vi "Group Memory.vi"(8 "error in (no error)":errorcluster, 9 "Group Initialization Set":T3[](array[typedef]), 10 "Group":string, 11 "Method":T5) -> (0 "error out":errorcluster, 1 "Group Indices Out":T4[](array[typedef]), 2 "Tag Sets Out":T1[](array[typedef]), 3 "Tags/Groups Out":string[](array[string]))   [LabVIEW 2016, in "CVT.lvlib" / "Current Value Table.lvlib"]
doc: "This VI stores references to the indices of every tag in each group, sorted by data type."
uses:
  <vilib>/NI/Current Value Table/Current Value Table.lvlib
  <vilib>/NI/Current Value Table/FGVs/Group Memory Methods.ctl
  <vilib>/NI/Current Value Table/Type Defs/Typed Index Set.ctl
  <vilib>/NI/Current Value Table/Type Defs/Data Types.ctl
  <vilib>/NI/Current Value Table/Type Defs/Group Initialization set.ctl
  <vilib>/NI/Current Value Table/Type Defs/Typed Name Set.ctl
  <vilib>/NI/Current Value Table/Errors/Generate Error.vi
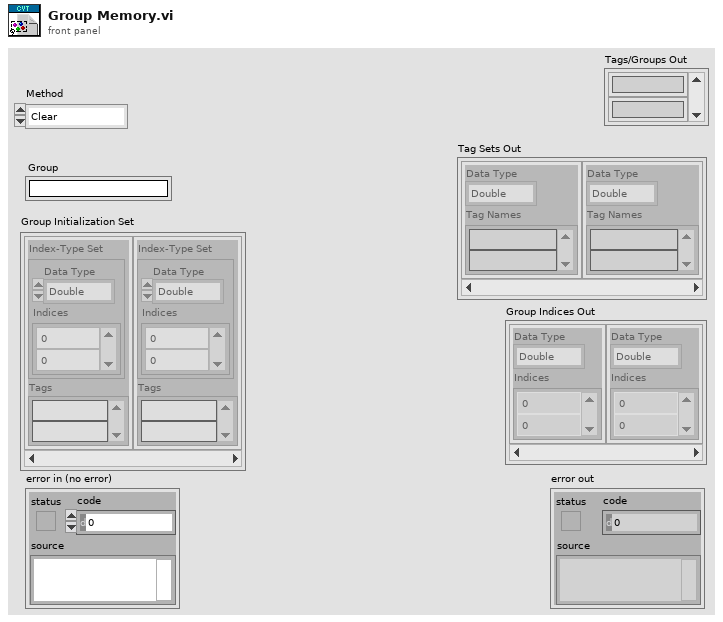
[diagram p1: front panel]
types:
  T1 = typedef "CVT.lvlib/Current Value Table.lvlib/Typed Name Set.ctl" = cluster{"Data Type":T2, "Tag Names":string[]}
  T2 = typedef "CVT.lvlib/Current Value Table.lvlib/Data Types.ctl" = enum16{"Double", "Single", "I64", "I32", "I16", "I8", "U64", "U32", "U16", "U8", "String", "Boolean", "Array of U8", "Array of U16", "Array of U32", "Array of U64", "Array of I64", "Array of I32", "Array of I16", "Array of I8", "Array of Double", "Array of Single", "Array of Boolean", "Array of String"}
  T3 = typedef "CVT.lvlib/Current Value Table.lvlib/Group Initialization set.ctl" = cluster{"Index-Type Set":T4, "Tags":string[]}
  T4 = typedef "CVT.lvlib/Current Value Table.lvlib/Typed Index Set.ctl" = cluster{"Data Type":T2, "Indices":i32[]}
  T5 = typedef "CVT.lvlib/Current Value Table.lvlib/Group Memory Methods.ctl" = enum16{"Clear", "Read Indices in Group", "List Groups", "List Tags by Type", "List Tags", "Delete Group", "Check Group Existence", "Create Group"}
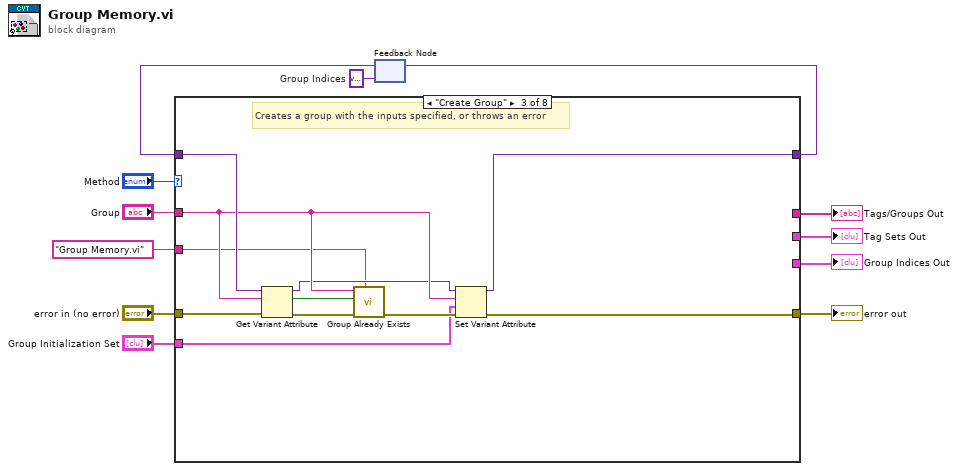
[diagram p0: block diagram]
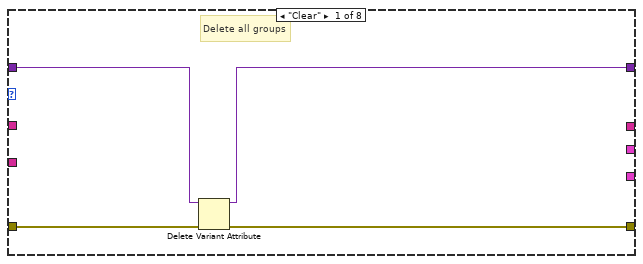
[diagram p2: hidden frame]
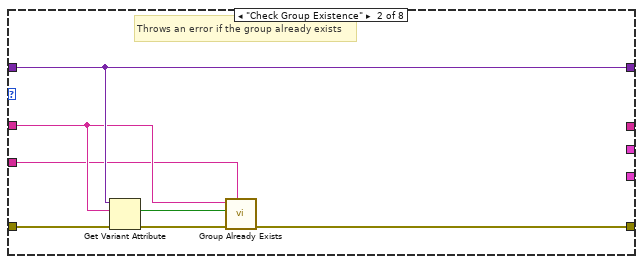
[diagram p3: hidden frame]
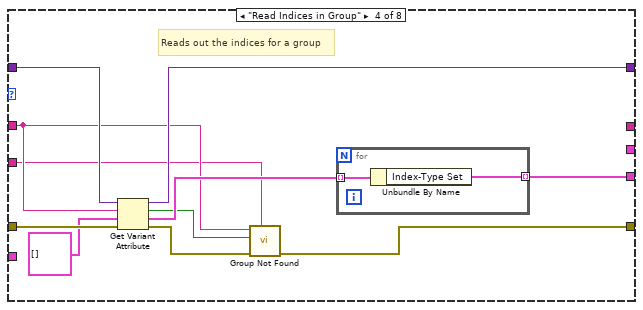
[diagram p4: hidden frame]
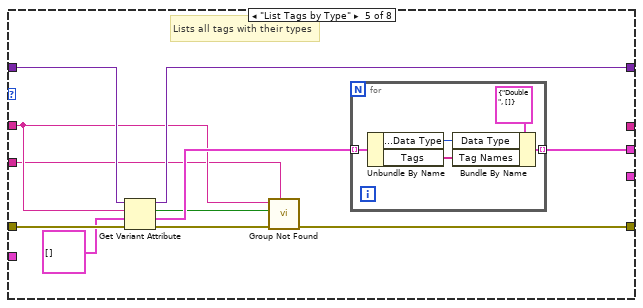
[diagram p5: hidden frame]
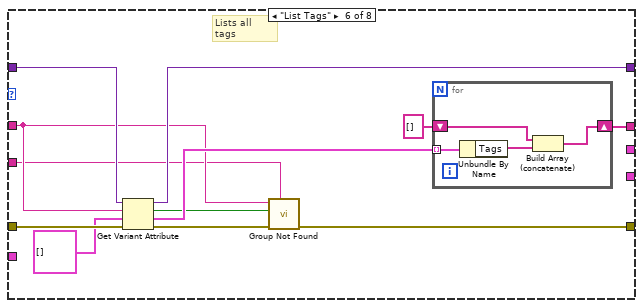
[diagram p6: hidden frame]
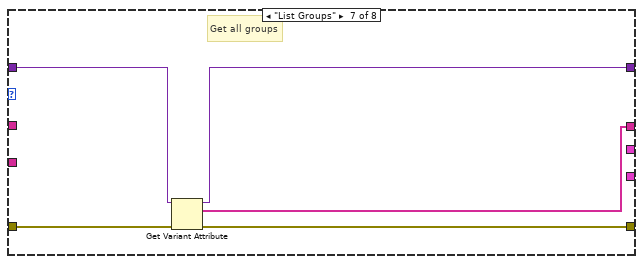
[diagram p7: hidden frame]
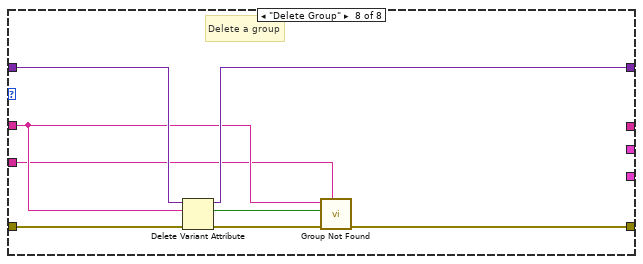
[diagram p8: hidden frame]
diagram:
  w12 = variant  # Group Indices
  n1 = feedback #1(w12) -> (w9:variant)
  n2 = case shown="\"Create Group\"" "Method" {
    tunnel: "Group" -> [_ w19 w28 w37 w50 w66 _ w86]
    tunnel: w9 -> [w14 w20 w29 w43 w57 w74 w82 w91]
    tunnel: [w13 w20 w34 w44 w56 w73 w81 w90] -> w8
    tunnel: "error in (no error)" -> [w16 w23 w33 w45 w58 w75 w84 w92]
    tunnel: [w15 w21 w30 w38 w51 w67 w83 w88] -> w6
    tunnel: [_ _ _ w40 _ _ _ _] -> w5
    tunnel: "Group Initialization Set" -> [_ _ w26 _ _ _ _ _]
    tunnel: [_ _ _ _ w53 _ _ _] -> w3
    tunnel: [_ _ _ _ _ w70 w80 _] -> w2
    tunnel: "Group Memory.vi" ("caller name") -> [_ w17 w24 w35 w48 w64 _ w85]
    frame "Clear" {
      # "Delete all groups"
      n3 = Delete Variant Attribute(4:w16, 7:w14) -> (0:w15:errorcluster, 3:w13:variant)  [unwired: 1 in, 1 out]
    }
    frame "Check Group Existence" {
      # "Throws an error if the group already exists"
      n4 = Get Variant Attribute(Variant=w20, name=w19, error in=w23) -> (found=w18:bool, error out=w22:errorcluster)  [unwired: 1 in, 2 out]
      n5 = call <vilib>:"Group Already Exists.vi"("caller name"=w17, "error in (no error)"=w22, "found?"=w18, "Group"=w19) -> ("error out"=w21:errorcluster)  [unwired: 7 in]
    }
    frame "Create Group" {
      # "Creates a group with the inputs specified, or throws an error"
      n6 = Get Variant Attribute(Variant=w29, name=w28, error in=w33) -> (duplicate Variant=w27:variant, found=w25:bool, error out=w32:errorcluster)  [unwired: 1 in, 1 out]
      n7 = call <vilib>:"Group Already Exists.vi"("caller name"=w24, "error in (no error)"=w32, "found?"=w25, "Group"=w28) -> ("error out"=w31:errorcluster)  [unwired: 7 in]
      n8 = Set Variant Attribute(Variant=w27, name=w28, value=w26, error in=w31) -> (Variant out=w34:variant, error out=w30:errorcluster)  [unwired: 1 out]
    }
    frame "Read Indices in Group" {
      # "Reads out the indices for a group"
      n9 = Get Variant Attribute(Variant=w43, name=w37, default value (empty Variant)=T3[] [] ("Group Initialization Set"), error in=w45) -> (duplicate Variant=w44:variant, found=w36:bool, value=w41:T3[], error out=w39:errorcluster)
      n10 = call <vilib>:"Group Not Found.vi"("caller name"=w35, "error in (no error)"=w39, "found?"=w36, "Group"=w37) -> ("error out"=w38:errorcluster)  [unwired: 7 in]
      n11 = for {
        tunnel: w41 -> [w47] mode=indexing
        tunnel: [w46] -> w40 mode=indexing
        n12 = Unbundle By Name(w47) -> ("Index-Type Set"=w46:T4)
      }
    }
    frame "List Tags by Type" {
      # "Lists all tags with their types"
      n13 = Get Variant Attribute(Variant=w57, name=w50, default value (empty Variant)=T3[] [] ("Group Initialization Set"), error in=w58) -> (duplicate Variant=w56:variant, found=w49:bool, value=w54:T3[], error out=w52:errorcluster)
      n14 = call <vilib>:"Group Not Found.vi"("caller name"=w48, "error in (no error)"=w52, "found?"=w49, "Group"=w50) -> ("error out"=w51:errorcluster)  [unwired: 7 in]
      n15 = for {
        tunnel: w54 -> [w63] mode=indexing
        tunnel: [w59] -> w53 mode=indexing
        n16 = Unbundle By Name(w63) -> ("Index-Type Set.Data Type"=w60:T2, "Tags"=w61:string[])
        n17 = Bundle By Name(cluster=T1 {"Data Type"=enum."Double", "Tag Names"=[]} ("Name Type Set"), "Data Type"=w60, "Tag Names"=w61) -> (w59:T1)
      }
    }
    frame "List Tags" {
      # "Lists all tags"
      n18 = Get Variant Attribute(Variant=w74, name=w66, default value (empty Variant)=T3[] [] ("Group Initialization Set"), error in=w75) -> (duplicate Variant=w73:variant, found=w65:bool, value=w71:T3[], error out=w68:errorcluster)
      n19 = call <vilib>:"Group Not Found.vi"("caller name"=w64, "error in (no error)"=w68, "found?"=w65, "Group"=w66) -> ("error out"=w67:errorcluster)  [unwired: 7 in]
      n20 = for {
        tunnel: w71 -> [w79] mode=indexing
        shift-right: [w77] -> w70
        shift-left: string[] [] -> [w76]
        n21 = Unbundle By Name(w79) -> ("Tags"=w78:string[])
        n22 = Build Array (concatenate)(w76, w78) -> (w77:string[])
      }
    }
    frame "List Groups" {
      # "Get all groups"
      n23 = Get Variant Attribute(Variant=w82, error in=w84) -> (duplicate Variant=w81:variant, names=w80:string[], error out=w83:errorcluster)  [unwired: 2 in, 1 out]
    }
    frame "Delete Group" {
      # "Delete a group"
      n24 = Delete Variant Attribute(4:w92, 6:w86, 7:w91) -> (0:w89:errorcluster, 2:w87:bool, 3:w90:variant)
      n25 = call <vilib>:"Group Not Found.vi"("caller name"=w85, "error in (no error)"=w89, "found?"=w87, "Group"=w86) -> ("error out"=w88:errorcluster)  [unwired: 7 in]
    }
  }
  "error out" <- w6
  "Group Indices Out" <- w5
  "Tag Sets Out" <- w3
  "Tags/Groups Out" <- w2
  n26 = feedback-in #1(w8) -> ()
